vi "Parallel Mode Circuit Number of Fourth Secondary Channel Read Array.vi"(8 "error in":errorcluster, 11 "Parallel Mode Channels In":refnum<class "Parallel Mode Channels.lvclass">) -> (0 "error out":errorcluster, 1 "Changed or First Call?":bool, 2 "Fourth Secondary Channel Circuit Number CTL":i32[](array[numeric]), 3 "Parallel Mode Channels Out":refnum<class "Parallel Mode Channels.lvclass">)   [LabVIEW 2023, in "Parallel Mode Channels.lvclass"]
uses:
  Parallel Mode Channels.lvclass
  Parallel Mode Channels.lvclass/Parallel Mode Channels.ctl
  <vilib>/ADAS Replay HIL/Channels/Tag Wrapper/Polymorphic/Read Channel (I32).vi
  6f7822f7-a431-4576-be95-9c573916d336.vi
  <vilib>/ADAS Replay HIL/Channels/Tag Wrapper/Polymorphic/Read Channel (I32).vi/b2f764de-0c1e-4784-a155-687fc995a684.vi
  <vilib>/ADAS Replay HIL/Channels/Tag Wrapper/Polymorphic/Read Channel (I32).vi/b2f764de-0c1e-4784-a155-687fc995a684.vi/c28b0ead-42ad-4072-80a2-aca7f2bd7ce3.vi
  <vilib>/ADAS Replay HIL/Channels/Tag Wrapper/Polymorphic/Read Channel (I32).vi/b2f764de-0c1e-4784-a155-687fc995a684.vi/219d0231-d98b-4193-b5cc-84f90e3c9091.vi
  <vilib>/ADAS Replay HIL/Channels/Tag Wrapper/Tag Wrapper.lvlib
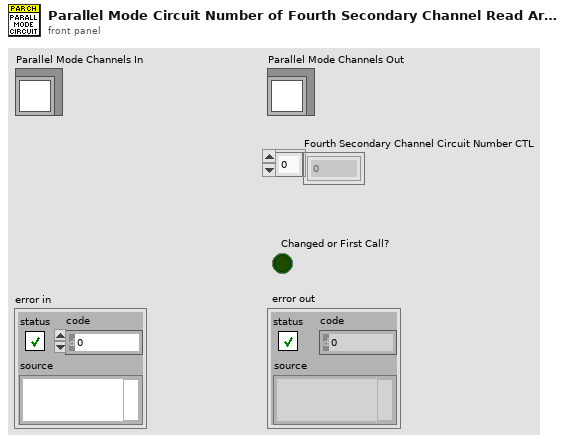
[diagram p1: front panel]
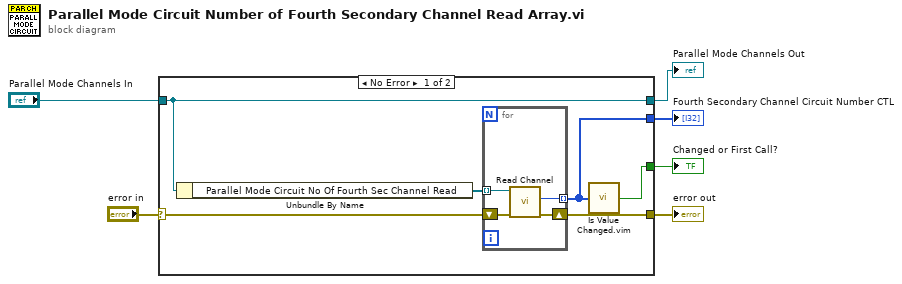
[diagram p0: block diagram]
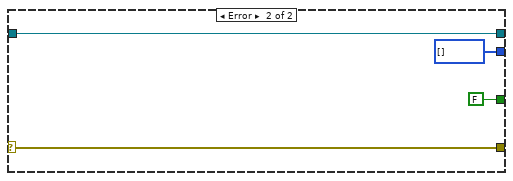
[diagram p2: hidden frame]
diagram:
  n1 = case shown="No Error" "error in" {
    selector: "error in" -> [w12 w20]
    tunnel: [w11 w20] -> w5
    tunnel: [w7 w19] -> w2
    tunnel: "Parallel Mode Channels In" -> [w7 w19]
    tunnel: [w10 i32[] []] -> w1
    tunnel: [w9 FALSE ("changed or first call?")] -> w4
    frame No Error {
      n2 = Unbundle By Name(w7) -> ("Parallel Mode Circuit No Of Fourth Sec Channel Read"=w8:refnum<k21>[])
      n3 = for {
        tunnel: [w14] -> w10 mode=indexing
        shift-right: [w15] -> w11
        shift-left: w12 -> [w16]
        tunnel: w8 -> [w13] mode=indexing
        n4 = call-poly <vilib>:"Read Channel.vi"("error in"=w16, "ADAS HIL Channel in"=w13) -> ("error out"=w15:errorcluster, "Value out"=w14:i32)  [unwired: 6 in, 2 out]
      }
      n5 = call "Is Value Changed.vim"("value"=w10) -> ("changed or first call?"=w9:bool)
    }
    frame Error {
    }
  }
  "error out" <- w5
  "Changed or First Call?" <- w4
  "Parallel Mode Channels Out" <- w2
  "Fourth Secondary Channel Circuit Number CTL" <- w1
